vi "Simulated LIDAR - compute r0 and phi.vi"(2 "y2":dbl, 3 "x2":dbl, 4 "y1":dbl, 5 "x1":dbl) -> (0 "phi":dbl, 1 "r0":dbl)   [LabVIEW 2017]
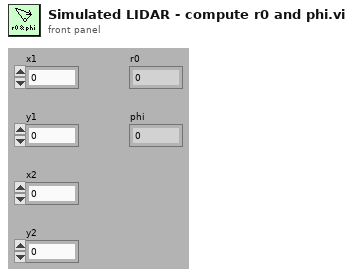
[diagram p1: front panel]
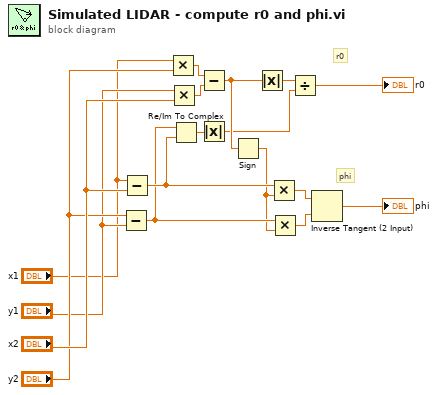
[diagram p0: block diagram]
diagram:
  # "phi"
  # "r0"
  n1 = Subtract(x="y2", y="y1") -> (x-y=w11:dbl)
  n2 = Subtract(x="x1", y="x2") -> (x-y=w12:dbl)
  n3 = Multiply(x="x1", y="y2") -> (x*y=w6:dbl)
  n4 = Multiply(x="y1", y="x2") -> (x*y=w5:dbl)
  n5 = Re/Im To Complex(1:w12, 2:w11) -> (0:w1:cdb)
  n6 = Subtract(x=w6, y=w5) -> (x-y=w9:dbl)
  n7 = Absolute Value(x=w1) -> (abs(x)=w8:dbl)
  n8 = Sign(1:w9) -> (0:w10:dbl)
  n9 = Absolute Value(x=w9) -> (abs(x)=w7:dbl)
  n10 = Multiply(x=w12, y=w10) -> (x*y=w13:dbl)
  n11 = Multiply(x=w11, y=w10) -> (x*y=w14:dbl)
  n12 = Divide(x=w7, y=w8) -> (x/y=→"r0":dbl)
  n13 = Inverse Tangent (2 Input)(1:w14, 2:w13) -> (0:→"phi":dbl)
